vi "Initialization (SILAR).vi"(8 "Error In":errorcluster, 11 "Arduino Resource In":T1={"VISA resource"="", "Board Type"=enum."Uno", "Connection Type"=enum."USB / Serial", "Bytes Per Packet (15)"=15}) -> (0 "Error Out":errorcluster, 3 "Arduino Resource Out":T1={"VISA resource"="", "Board Type"=enum."Uno", "Connection Type"=enum."USB / Serial", "Bytes Per Packet (15)"=15})   [LabVIEW 2016]
uses:
  <vilib>/LabVIEW Interface for Arduino/Type Defs/Arduino Resource.ctl
  <vilib>/LabVIEW Interface for Arduino/Type Defs/Board Type.ctl
  <vilib>/LabVIEW Interface for Arduino/Type Defs/Pin Mode.ctl
  <vilib>/LabVIEW Interface for Arduino/LabVIEW Interface for Arduino.lvlib
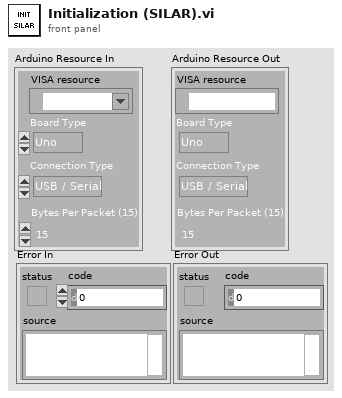
[diagram p1: front panel]
types:
  T1 = typedef "LabVIEW Interface for Arduino.lvlib/Arduino Resource.ctl" = cluster{"VISA resource":refnum<visa-resource-name>, "Board Type":T2, "Connection Type":enum8{"USB / Serial"}, "Bytes Per Packet (15)":u8}
  T2 = typedef "LabVIEW Interface for Arduino.lvlib/Board Type.ctl" = enum16{"Uno", "Dimuelanove w/Atmega 328", "Mega 2560"}
  T3 = typedef "LabVIEW Interface for Arduino.lvlib/Pin Mode.ctl" = enum8{"Input", "Output"}
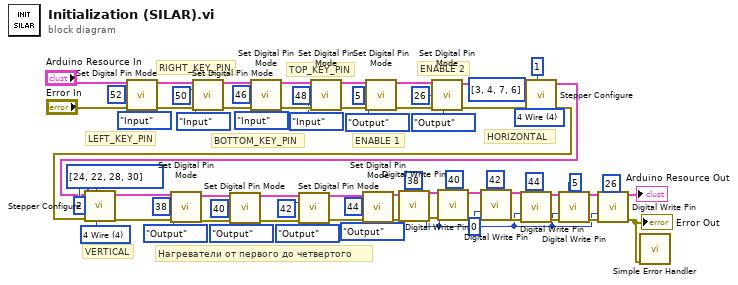
[diagram p0: block diagram]
diagram:
  w14 = u8 4 items=["2 Wire (Pulse & Direction)"=1, "2 Wire"=2, "4 Wire"=4, "EasyDriver"=6, "AF Motor Shield (Stepper 1 & 2 Only)"=5] ("Control Method")
  w3 = u8 0 ("Value (0)")
  w55 = u8 4 items=["2 Wire (Pulse & Direction)"=1, "2 Wire"=2, "4 Wire"=4, "EasyDriver"=6, "AF Motor Shield (Stepper 1 & 2 Only)"=5] ("Control Method")
  # "HORIZONTAL"
  # "Нагреватели от первого до четвертого"
  # "ENABLE 2"
  # "ENABLE 1"
  # "VERTICAL"
  # "RIGHT_KEY_PIN"
  # "TOP_KEY_PIN"
  # "BOTTOM_KEY_PIN"
  # "LEFT_KEY_PIN"
  n1 = call <vilib>:"Set Digital Pin Mode.vi"("Arduino Resource"="Arduino Resource In", "Digital I/O Pin"=u8 52, "Pin Mode (Input)"=Pin_Mode."Input", "error in"="Error In") -> ("Arduino Resource"=w71:T1, "error out"=w68:errorcluster)  [unwired: 10 in]
  n2 = call <vilib>:"Set Digital Pin Mode.vi"("Arduino Resource"=w71, "Digital I/O Pin"=u8 50, "Pin Mode (Input)"=Pin_Mode."Input", "error in"=w68) -> ("Arduino Resource"=w70:T1, "error out"=w67:errorcluster)  [unwired: 10 in]
  n3 = call <vilib>:"Set Digital Pin Mode.vi"("Arduino Resource"=w70, "Digital I/O Pin"=u8 46, "Pin Mode (Input)"=Pin_Mode."Input", "error in"=w67) -> ("Arduino Resource"=w69:T1, "error out"=w66:errorcluster)  [unwired: 10 in]
  n4 = call <vilib>:"Set Digital Pin Mode.vi"("Arduino Resource"=w69, "Digital I/O Pin"=u8 48, "Pin Mode (Input)"=Pin_Mode."Input", "error in"=w66) -> ("Arduino Resource"=w17:T1, "error out"=w50:errorcluster)  [unwired: 10 in]
  n5 = call <vilib>:"Set Digital Pin Mode.vi"("Arduino Resource"=w17, "Digital I/O Pin"=u8 5, "Pin Mode (Input)"=Pin_Mode."Output", "error in"=w50) -> ("Arduino Resource"=w48:T1, "error out"=w49:errorcluster)  [unwired: 10 in]
  n6 = call <vilib>:"Set Digital Pin Mode.vi"("Arduino Resource"=w48, "Digital I/O Pin"=u8 26, "Pin Mode (Input)"=Pin_Mode."Output", "error in"=w49) -> ("Arduino Resource"=w13:T1, "error out"=w12:errorcluster)  [unwired: 10 in]
  n7 = call <vilib>:"Stepper Configure.vi"("Control Method"=w14, "Stepper #"=u8 1, "error in"=w12, "Stepper Pins"=u8[] [3, 4, 7, 6], "Arduino Resource"=w13) -> ("error out"=w10:errorcluster, "Arduino Resource Out"=w11:T1)  [unwired: 5 in]
  n8 = call <vilib>:"Stepper Configure.vi"("Control Method"=w55, "Stepper #"=u8 2, "error in"=w10, "Stepper Pins"=u8[] [24, 22, 28, 30], "Arduino Resource"=w11) -> ("error out"=w30:errorcluster, "Arduino Resource Out"=w31:T1)  [unwired: 5 in]
  n9 = call <vilib>:"Set Digital Pin Mode.vi"("Arduino Resource"=w31, "Digital I/O Pin"=u8 38, "Pin Mode (Input)"=Pin_Mode."Output", "error in"=w30) -> ("Arduino Resource"=w37:T1, "error out"=w32:errorcluster)  [unwired: 10 in]
  n10 = call <vilib>:"Set Digital Pin Mode.vi"("Arduino Resource"=w37, "Digital I/O Pin"=u8 40, "Pin Mode (Input)"=Pin_Mode."Output", "error in"=w32) -> ("Arduino Resource"=w36:T1, "error out"=w33:errorcluster)  [unwired: 10 in]
  n11 = call <vilib>:"Set Digital Pin Mode.vi"("Arduino Resource"=w36, "Digital I/O Pin"=u8 42, "Pin Mode (Input)"=Pin_Mode."Output", "error in"=w33) -> ("Arduino Resource"=w35:T1, "error out"=w34:errorcluster)  [unwired: 10 in]
  n12 = call <vilib>:"Set Digital Pin Mode.vi"("Arduino Resource"=w35, "Digital I/O Pin"=u8 44, "Pin Mode (Input)"=Pin_Mode."Output", "error in"=w34) -> ("Arduino Resource"=w18:T1, "error out"=w19:errorcluster)  [unwired: 10 in]
  n13 = call <vilib>:"Digital Write Pin.vi"("Arduino Resource"=w18, "Digital I/O Pin (0)"=u8 38, "Value (0)"=w3, "error in"=w19) -> ("Arduino Resource"=w25:T1, "error out"=w24:errorcluster)  [unwired: 10 in]
  n14 = call <vilib>:"Digital Write Pin.vi"("Arduino Resource"=w25, "Digital I/O Pin (0)"=u8 40, "Value (0)"=w3, "error in"=w24) -> ("Arduino Resource"=w26:T1, "error out"=w27:errorcluster)  [unwired: 10 in]
  n15 = call <vilib>:"Digital Write Pin.vi"("Arduino Resource"=w26, "Digital I/O Pin (0)"=u8 42, "Value (0)"=w3, "error in"=w27) -> ("Arduino Resource"=w29:T1, "error out"=w28:errorcluster)  [unwired: 10 in]
  n16 = call <vilib>:"Digital Write Pin.vi"("Arduino Resource"=w29, "Digital I/O Pin (0)"=u8 44, "Value (0)"=w3, "error in"=w28) -> ("Arduino Resource"=w7:T1, "error out"=w4:errorcluster)  [unwired: 10 in]
  n17 = call <vilib>:"Digital Write Pin.vi"("Arduino Resource"=w7, "Digital I/O Pin (0)"=u8 5, "Value (0)"=w3, "error in"=w4) -> ("Arduino Resource"=w6:T1, "error out"=w5:errorcluster)  [unwired: 10 in]
  n18 = call <vilib>:"Digital Write Pin.vi"("Arduino Resource"=w6, "Digital I/O Pin (0)"=u8 26, "Value (0)"=w3, "error in"=w5) -> ("Arduino Resource"=→"Arduino Resource Out":T1, "error out"=w2:errorcluster)  [unwired: 10 in]
  "Error Out" <- w2
  n19 = call <vilib>:"Simple Error Handler.vi"("error in (no error)"=w2) -> ()  [unwired: 4 in, 5 out]
